vi "3-1.vi"(0 "x":dbl) -> (1 "正弦":dbl, 2 "余弦":dbl)   [LabVIEW 2017]
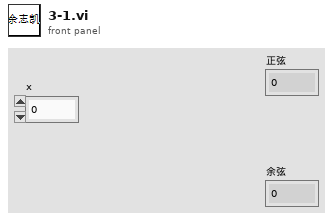
[diagram p1: front panel]
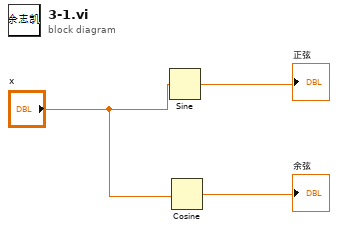
[diagram p0: block diagram]
diagram:
  n1 = Sine(x="x") -> (sin(x)=→"正弦":dbl)
  n2 = Cosine(x="x") -> (cos(x)=→"余弦":dbl)
